vi "Garbagio-AB_BC_Chopper_Single.vi"(8 "Decimate point":dbl=1e-10 format="%#_1f", 9 "Portion of data":cluster{dbl, dbl}(slide)={0.75, 0.25} scale=0.0..1.0, 10 "input IV CD":cluster{dbl[], dbl[]}(graph)={array[2480 elements], array[2480 elements]}, 11 "input IV AB":cluster{dbl[], dbl[]}(graph)={array[2480 elements], array[2480 elements]}) -> (2 "Chopped AB thing":cluster{dbl[], dbl[]}, 3 "Chopped BC thing":cluster{dbl[], dbl[]})   [LabVIEW 2016]
uses:
  <vilib>/Analysis/2dsp.llb/Decimate (single shot, DBL).vi
  <vilib>/Analysis/NI_AALPro.lvlib
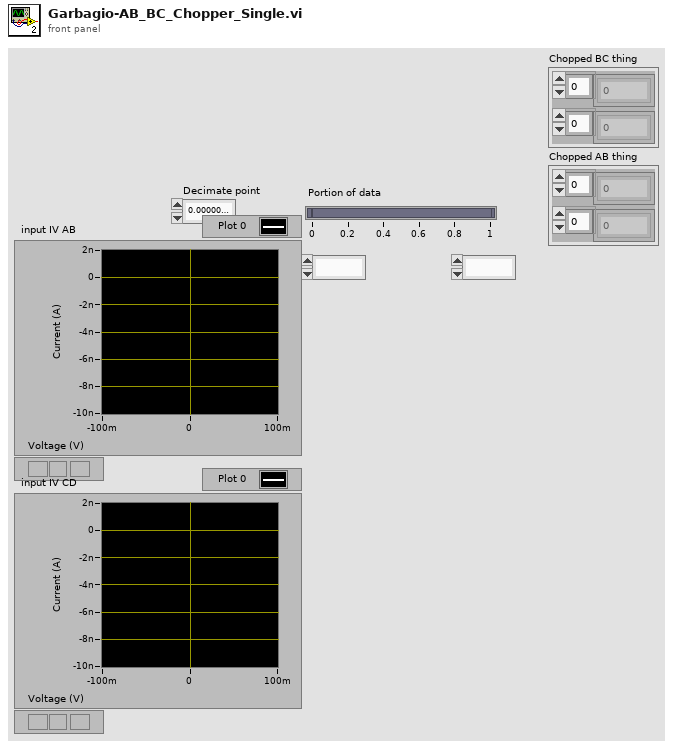
[diagram p1: front panel]
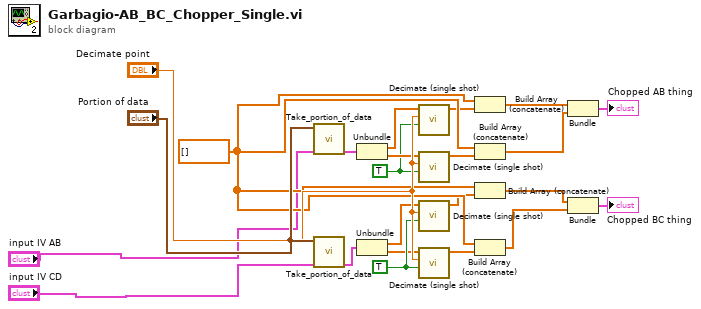
[diagram p0: block diagram]
diagram:
  w5 = TRUE ("averaging")
  w12 = TRUE ("averaging")
  w19 = dbl[] []
  n1 = call <userlib>:"Take_portion_of_data.vi"("input IV"="input IV AB", "Slide"="Portion of data") -> ("Output IV"=w11:cluster{dbl[], dbl[]})  [unwired: 5 in]
  n2 = call <userlib>:"Take_portion_of_data.vi"("input IV"="input IV CD", "Slide"="Portion of data") -> ("Output IV"=w6:cluster{dbl[], dbl[]})  [unwired: 5 in]
  n3 = Unbundle(w11) -> (w13:dbl[], w14:dbl[])
  n4 = Unbundle(w6) -> (w4:dbl[], w3:dbl[])
  n5 = call-poly <vilib>:"Decimate (single shot).vi"("averaging"=w12, "decimating factor"="Decimate point", "X"=w13) -> ("Decimated Array"=w10:dbl[])  [unwired: 7 in, 1 out]
  n6 = call-poly <vilib>:"Decimate (single shot).vi"("averaging"=w12, "decimating factor"="Decimate point", "X"=w14) -> ("Decimated Array"=w9:dbl[])  [unwired: 7 in, 1 out]
  n7 = call-poly <vilib>:"Decimate (single shot).vi"("averaging"=w5, "decimating factor"="Decimate point", "X"=w4) -> ("Decimated Array"=w7:dbl[])  [unwired: 7 in, 1 out]
  n8 = call-poly <vilib>:"Decimate (single shot).vi"("averaging"=w5, "decimating factor"="Decimate point", "X"=w3) -> ("Decimated Array"=w8:dbl[])  [unwired: 7 in, 1 out]
  n9 = Build Array (concatenate)(w19, w10) -> (w21:dbl[])
  n10 = Build Array (concatenate)(w19, w9) -> (w20:dbl[])
  n11 = Build Array (concatenate)(w19, w7) -> (w18:dbl[])
  n12 = Build Array (concatenate)(w19, w8) -> (w17:dbl[])
  n13 = Bundle(w21, w20) -> (→"Chopped AB thing":cluster{dbl[], dbl[]})  [unwired: 1 in]
  n14 = Bundle(w18, w17) -> (→"Chopped BC thing":cluster{dbl[], dbl[]})  [unwired: 1 in]
